vi "Untitled 5.vi"() -> ()   [LabVIEW 2019]
uses:
  <vilib>/userDefined/High Color/IMAQdx.ctl
  <vilib>/vision/driver/NI_Vision_Acquisition_Software.lvlib
panel:
  out "Time":dbl
  out "MaxVal":dbl
  out "Image":T1(plugin-control)
  out "BestZ":dbl
  in  "SafeZ":dbl
  in  "StartZ":dbl
  in  "ScanRange":dbl=0.4 format="%#_13g"
  in  "Camera":T2="cam1"
  in  "error in (no error)":errorcluster
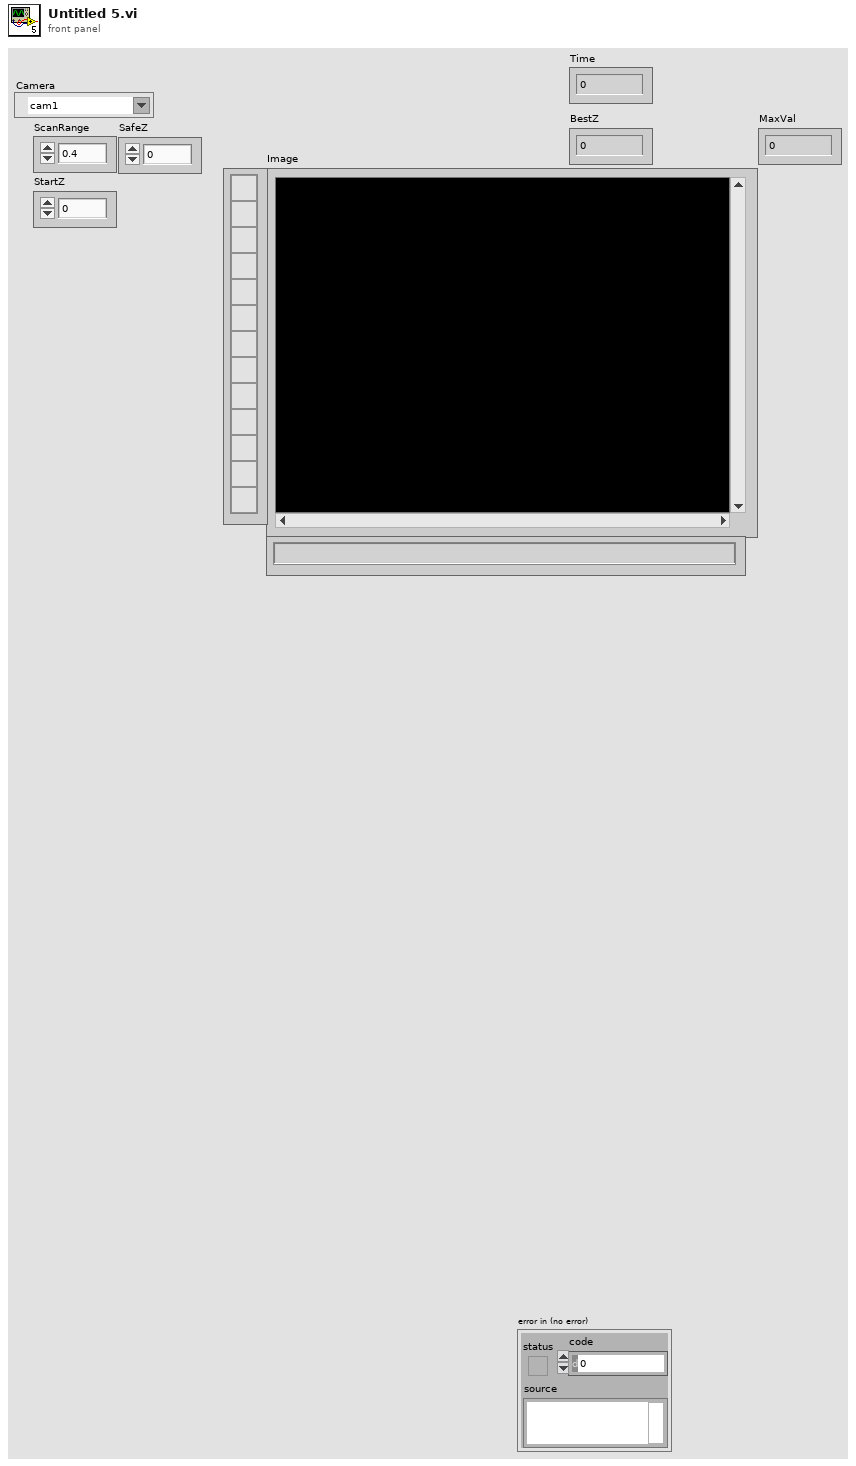
[diagram p1: front panel]
types:
  T1 = typedef "IMAQ Image.ctl" = refnum<image>
  T2 = typedef "IMAQdx.ctl" = refnum<k21>
  T3 = typedef "Image Type" = u32
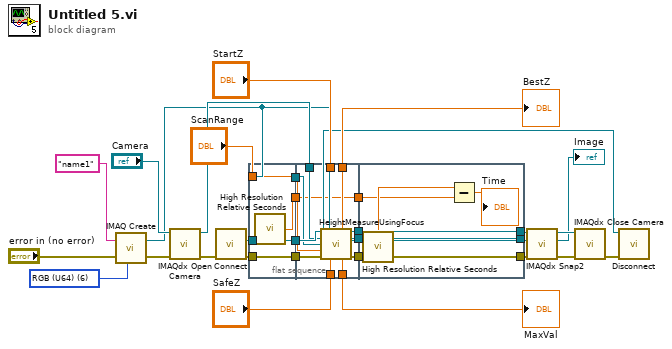
[diagram p0: block diagram]
diagram:
  w28 = T3 6 items=["Grayscale (U8)", "Grayscale (I16)", "Grayscale (SGL)", "Complex (CSG)", "RGB (U32)", "HSL (U32)", "RGB (U64)", "Grayscale (U16)"] ("Image Type")
  n1 = call "IMAQ Create"("Image Name"="name1" ("ImageName"), "Image Type"=w28, "error in (no error)"="error in (no error)") -> ("New Image"=w14:T1, "error out"=w30:errorcluster)  [unwired: 2 in]
  n2 = call <vilib>:"IMAQdx Open Camera.vi"("error in"=w30, "Session In"="Camera") -> ("error out"=w26:errorcluster, "Session Out"=w23:T2)  [unwired: 8 in]
  n3 = call "Connect.vi"("error in (no error)"=w26) -> ("error out"=w21:errorcluster, "controller"=w24:refnum<k24>)  [unwired: 9 in]
  n4 = flat-sequence {
    tunnel: w14 -> [w33]
    tunnel: w21 -> [w34]
    tunnel: "ScanRange" -> [w35]
    tunnel: w24 -> [w36]
    tunnel: [w36] -> w6
    tunnel: [w35] -> w5
    tunnel: [w34] -> w4
    tunnel: [w33] -> w3
    tunnel: [w32] -> w1
    tunnel: w23 -> [w48]
    tunnel: "StartZ" -> [w45]
    tunnel: [w44] -> w19
    tunnel: "SafeZ" -> [w42]
    tunnel: [w41] -> w16
    tunnel: [w43] -> w9
    tunnel: [w40] -> w8
    tunnel: [w38] -> w7
    tunnel: w6 -> [w49]
    tunnel: w5 -> [w47]
    tunnel: w4 -> [w46]
    tunnel: w3 -> [w39]
    tunnel: [w37] -> w2
    tunnel: w1 -> [w37]
    tunnel: [w53] -> w11
    tunnel: [w54] -> w15
    tunnel: [w55] -> w18
    tunnel: w9 -> [w55]
    tunnel: w8 -> [w54]
    tunnel: w7 -> [w53]
    tunnel: w2 -> [w51]
    frame #0 {
      n5 = call <vilib>:"High Resolution Relative Seconds.vi"() -> ("relative seconds"=w32:dbl)
    }
    frame #1 {
      n6 = call "HeightMeasureUsingFocus.vi"("controller in"=w49, "StartZ"=w45, "SessionIn"=w48, "ImageIn"=w39, "ScanRange"=w47, "error in (no error)"=w46, "SafeZ"=w42) -> ("BestZ"=w44:dbl, "controller out"=w43:refnum<k24>, "Session Out"=w40:T2, "MaxVal"=w41:dbl, "Error Out"=w38:errorcluster)  [unwired: 3 in, 1 out]
    }
    frame #2 {
      n7 = call <vilib>:"High Resolution Relative Seconds.vi"() -> ("relative seconds"=w52:dbl)
      n8 = Subtract(x=w52, y=w51) -> (x-y=→"Time":dbl)
    }
  }
  n9 = call <vilib>:"IMAQdx Snap2.vi"("error in"=w11, "Image In"=w14, "Session In"=w15) -> ("error out"=w10:errorcluster, "Image Out"=→"Image":T1, "Session Out"=w13:T2)  [unwired: 6 in]
  n10 = call <vilib>:"IMAQdx Close Camera.vi"("error in"=w10, "Session In"=w13) -> ("error out"=w25:errorcluster)  [unwired: 9 in]
  n11 = call "Disconnect.vi"("error in (no error)"=w25, "controller"=w18) -> ()  [unwired: 9 in, 1 out]
  "BestZ" <- w19
  "MaxVal" <- w16
